vi "Format Into Table.vi"(8 "error in (no error)":errorcluster, 11 "Statement in":refnum<class "Statement.lvclass">) -> (0 "error out":errorcluster, 3 "Table Row":string[][](array[string]))   [LabVIEW 2018, in "Statement.lvclass"]
uses:
  Statement.lvclass
  Statement.lvclass/Statement.ctl
  Transaction/Transaction.lvclass
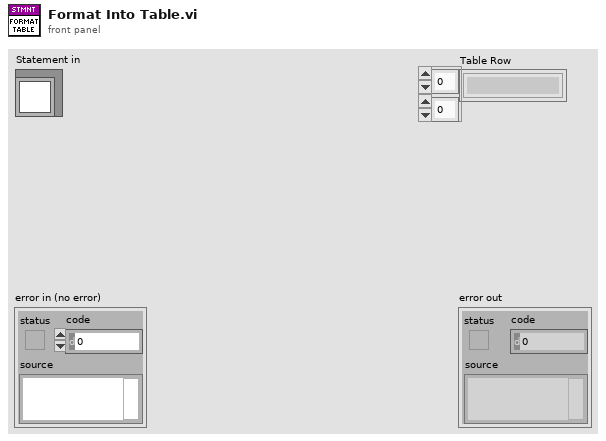
[diagram p1: front panel]
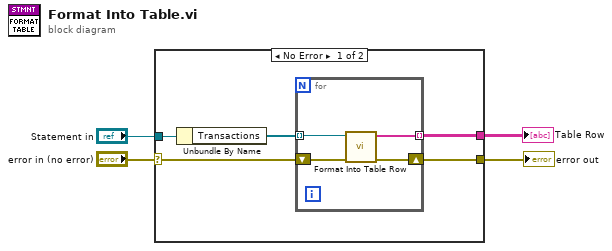
[diagram p0: block diagram]
diagram:
  n1 = case shown="No Error" "error in (no error)" {
    selector: "error in (no error)" -> [w7 w14]
    tunnel: [w6 w14] -> w3
    tunnel: "Statement in" -> [w9 _]
    tunnel: [w5 _] -> w1
    frame No Error {
      n2 = Unbundle By Name(w9) -> ("Transactions"=w8:refnum<class "Transaction.lvclass">[])
      n3 = for {
        tunnel: w8 -> [w13] mode=indexing
        tunnel: [w12] -> w5 mode=indexing
        shift-right: [w10] -> w6
        shift-left: w7 -> [w11]
        n4 = call "Format Into Table Row.vi"("error in (no error)"=w11, "Transaction in"=w13) -> ("error out"=w10:errorcluster, "Table Row"=w12:string[])  [unwired: 8 in]
      }
    }
    frame Error {
    }
  }
  "error out" <- w3
  "Table Row" <- w1
